vi "Array2Matrix_test.vi"(1 "Array":sgl[](array[numeric]), 2 "Header":string[](array[string])) -> (0 "Array2D":sgl[][](array[numeric]))   [LabVIEW 2021]
panel:
  out "Numeric":i32
  out "size of Array3":i32
  out "size(s)":i32[](array[numeric])
  out "Array3":sgl[](array[numeric])
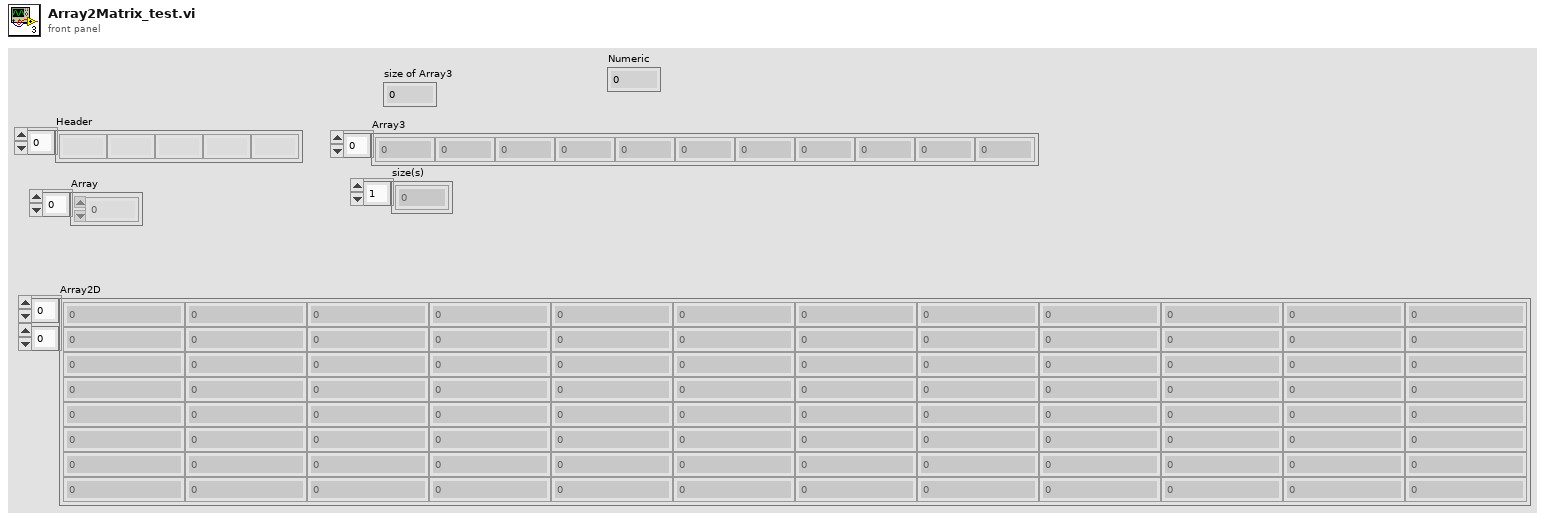
[diagram p1: front panel]
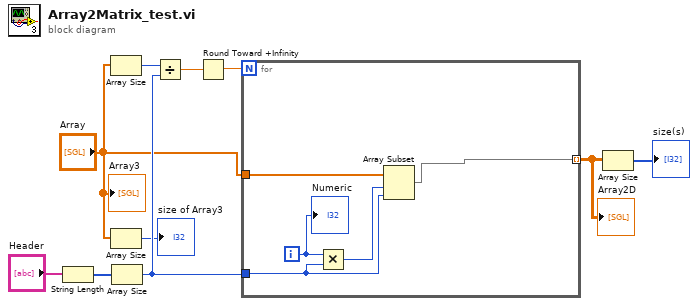
[diagram p0: block diagram]
diagram:
  n1 = String Length(string="Header") -> (length=w9:i32[])
  n2 = Array Size(array="Array") -> (size(s)=w4:i32)
  n3 = Array Size(array="Array") -> (size(s)=→"size of Array3":i32)
  n4 = Array Size(array=w9) -> (size(s)=w8:i32)
  n5 = Divide(x=w4, y=w8) -> (x/y=w10:dbl)
  n6 = Round Toward +Infinity(x=w10) -> (ceil(x): smallest int >= x=w7:dbl)
  n7 = for {
    N: w7 -> [_]
    tunnel: "Array" -> [w15]
    tunnel: w8 -> [w13]
    tunnel: [w11] -> w1 mode=indexing
    i -> [w12]
    n8 = Multiply(x=w12, y=w13) -> (x*y=w14:i32)
    n9 = Array Subset(array=w15, index=w14, length=w13) -> (w11:sgl[])
    "Numeric" <- w12
  }
  "Array2D" <- w1
  n10 = Array Size(array=w1) -> (size(s)=→"size(s)":i32[])
  "Array3" <- "Array"
